vi "Write Monitor controller configuration.vi"(8 "error in (no error)":errorcluster, 10 "Configuration":T1={"Update period"=-1.0, "Repeat times"=-1, "Open plot"=FALSE, "File defragment period"=-1.0, "Timestamp data points"=FALSE, "Re-plot rate limit"=0.95} {"Re-plot rate limit" format="%#_6ps"; "File defragment period" format="%#_6ps"; "Update period" min=0.01 max=100.0 format="%#_6ps"}, 11 "Monitor Controller in":refnum<class "Monitor Controller.lvclass">) -> (0 "error out":errorcluster, 3 "Monitor Controller out":refnum<class "Monitor Controller.lvclass">)   [LabVIEW 2018, in "Monitor Controller.lvclass"]
uses:
  Monitor Controller.lvclass
  C:/github/LabActor/Template Module/Template Module.lvclass
  Monitor Controller Configuration.ctl
  Template Module/Template Module.lvclass/Template Module.ctl
  Template Module/Write Configuration.vi
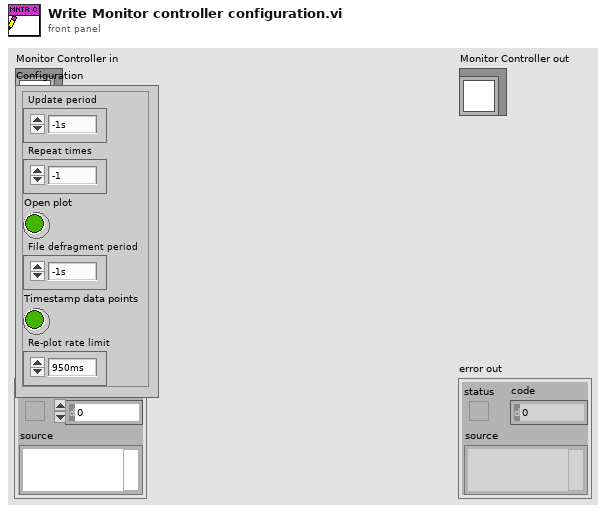
[diagram p1: front panel]
types:
  T1 = typedef "Monitor Controller Configuration.ctl" = cluster{"Update period":dbl, "Repeat times":i32, "Open plot":bool, "File defragment period":dbl, "Timestamp data points":bool, "Re-plot rate limit":dbl}
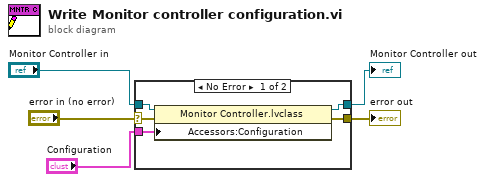
[diagram p0: block diagram]
diagram:
  n1 = case shown="No Error" "error in (no error)" {
    selector: "error in (no error)" -> [w7 w11]
    tunnel: [w6 w11] -> w4
    tunnel: [w9 w12] -> w2
    tunnel: "Monitor Controller in" -> [w10 w12]
    tunnel: "Configuration" -> [w8 _]
    frame No Error {
      n2 = property class="Monitor Controller.lvclass"(reference=w10, error in=w7, "Accessors:Configuration"=w8) -> (reference out=w9:refnum<class "Monitor Controller.lvclass">, error out=w6:errorcluster)
    }
    frame Error {
    }
  }
  "error out" <- w4
  "Monitor Controller out" <- w2
